vi "Minimal Error to String.vi"(8 "error in (no error)":errorcluster) -> (0 "String":string)   [LabVIEW 2020, in "NI_WFCN.lvlib"]
doc: "Formats an Error Cluster into a string, quickly."
uses:
  <vilib>/net/WFCN/NI_WFCN.lvlib
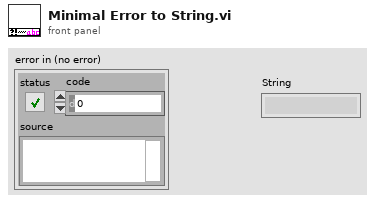
[diagram p1: front panel]
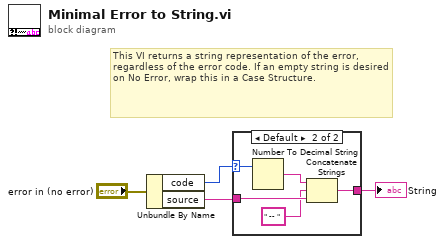
[diagram p0: block diagram]
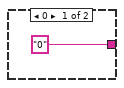
[diagram p2: hidden frame]
diagram:
  # "This VI returns a string representation of the error, regardless of the error code. If an empty string is desired on No Error, wrap this in a Case Structure."
  n1 = Unbundle By Name("error in (no error)") -> ("code"=w3:i32, "source"=w1:string)
  n2 = case shown="Default" w3 {
    selector: w3 -> [_ w7]
    tunnel: ["0" w9] -> w2
    tunnel: w1 -> [_ w10]
    frame 0 {
    }
    frame Default {
      n3 = Number To Decimal String(number=w7) -> (decimal integer string=w6:string)  [unwired: 1 in]
      n4 = Concatenate Strings(w6, " -- " ("string"), w10) -> (w9:string)
    }
  }
  "String" <- w2
